vi "FP pivot the boat.vi"(1 "Heading":dbl min=0.0 max=360.0 step=1.0, 2 "Image Pixels (U32)":u32[][](array[numeric])) -> (0 "Image pixels\nOut":u32[][](array[numeric]))   [LabVIEW 2014]
doc: "This vi accepts a color image array and a desired absolute boat heading. It rotates the boat image and return the new color image array."
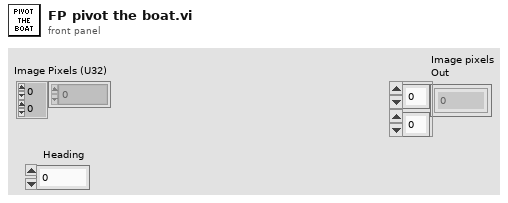
[diagram p1: front panel]
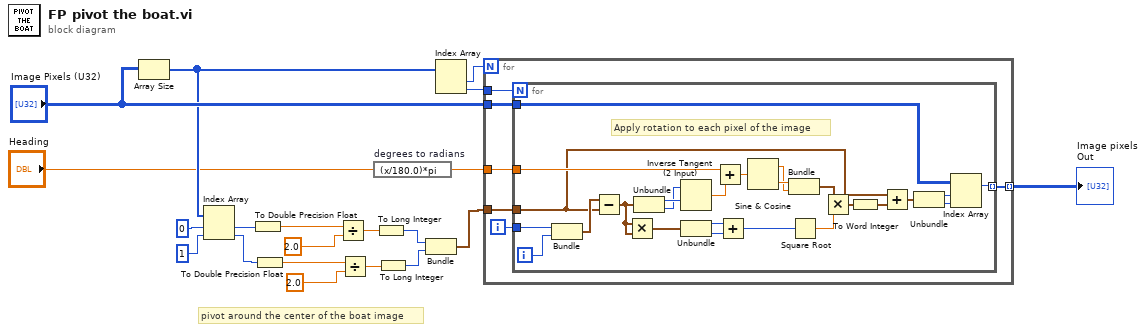
[diagram p0: block diagram]
diagram:
  # "pivot around the center of the boat image"
  n1 = Array Size(array="Image Pixels (U32)") -> (size(s)=w3:i32[])
  n2 = Index Array(array=w3, index #1=0 ("index"), index #2=1 ("index")) -> (element #1=w12:i32, element #2=w8:i32)
  n3 = To Double Precision Float(number=w12) -> (double precision float=w11:dbl)
  n4 = To Double Precision Float(number=w8) -> (double precision float=w9:dbl)
  n5 = Divide(x=w11, y=2.0) -> (x/y=w7:dbl)
  n6 = Divide(x=w9, y=2.0) -> (x/y=w6:dbl)
  n7 = expression code="(x/180.0)*pi" "degrees to radians"("Heading") -> (w20:dbl)
  n8 = To Long Integer(number=w7) -> (32bit integer=w5:i32)
  n9 = To Long Integer(number=w6) -> (32bit integer=w4:i32)
  n10 = Bundle(w5, w4) -> (w2:cluster{i32, i32})  [unwired: 1 in]
  n11 = Index Array(array=w3) -> (element #1=w18:i32, element #2=w19:i32)  [unwired: 2 in]
  n12 = for {
    N: w18 -> [_]
    tunnel: w19 -> [w25]
    tunnel: w2 -> [w24]
    tunnel: w20 -> [w23]
    tunnel: "Image Pixels (U32)" -> [w22]
    tunnel: [w21] -> w16 mode=indexing
    i -> [w26]
    n13 = for {
      N: w25 -> [_]
      tunnel: w26 -> [w51]
      tunnel: w24 -> [w29]
      tunnel: w23 -> [w40]
      tunnel: w22 -> [w30]
      tunnel: [w28] -> w21 mode=indexing
      i -> [w50]
      # "Apply rotation to each pixel of the image"
      n14 = Bundle(w51, w50) -> (w49:cluster{i32, i32})  [unwired: 1 in]
      n15 = Subtract(x=w49, y=w29) -> (x-y=w44:cluster{i32, i32})
      n16 = Multiply(x=w44, y=w44) -> (x*y=w48:cluster{i32, i32})
      n17 = Unbundle(w44) -> (w43:i32, w42:i32)
      n18 = Inverse Tangent (2 Input)(1:w43, 2:w42) -> (0:w41:dbl)
      n19 = Unbundle(w48) -> (w47:i32, w46:i32)
      n20 = Add(x=w40, y=w41) -> (x+y=w39:dbl)
      n21 = Add(x=w47, y=w46) -> (x+y=w45:i32)
      n22 = Sine & Cosine(0:w39) -> (1:w37:dbl, 2:w38:dbl)
      n23 = Bundle(w38, w37) -> (w36:cluster{dbl, dbl})  [unwired: 1 in]
      n24 = Square Root(x=w45) -> (sqrt(x)=w35:dbl)
      n25 = Multiply(x=w36, y=w35) -> (x*y=w34:cluster{dbl, dbl})
      n26 = To Word Integer(number=w34) -> (16bit integer=w33:cluster{i16, i16})
      n27 = Add(x=w29, y=w33) -> (x+y=w27:cluster{i32, i32})
      n28 = Unbundle(w27) -> (w32:i32, w31:i32)
      n29 = Index Array(array=w30, index (row)=w32, index (col)=w31) -> (element=w28:u32)
    }
  }
  "Image pixels\nOut" <- w16
